vi "PID_velocity.vi"() -> ()   [LabVIEW 2014]
uses:
  <vilib>/FPGAPlugInAG/cRIO-9068/niLvFpga_Open_cRIO-9068.vi
  <vilib>/rvi/interface/common/dynamic/niFpgaDynamicAddResources.vi
  <vilib>/Utility/error.llb/Error Cluster From Error Code.vi
  <vilib>/rvi/errors/niLvFpgaAdjustHostInterfaceError.vi
  <vilib>/addons/control/pid/pid.llb/PID (DBL).vi
  <vilib>/FPGAPlugInAG/Dynamic/niLvFpga_Close_Dynamic.vi
  <vilib>/rvi/interface/nirviOpenFPGA/nirviOpenFPGA.xnode
  FPGA Bitfiles/Motortest_FPGATarget_test6auto_Jx62XASY7Q8.lvbitx
  <vilib>/rvi/interface/nirviReadWriteControl/nirviReadWriteControl.xnode
  <vilib>/rvi/interface/nirviCloseFPGA/nirviCloseFPGA.xnode
  NiFpgaLv.dll
  <vilib>/rvi/interface/Simulation/niFpgaSimulationCallBeginRW.vi
  <vilib>/addons/control/pid/NI_PID_pid.lvlib
panel:
  out "Duty Cycle":dbl[](graph)
  out "Duty Cycle":dbl(slide) scale=0.0..1.0
  out "Error":dbl(slide) scale=0.0..50.0
  out "Velocity":sgl[](graph)
  out "Duty Cycle":dbl format="%.2f"
  in  "output range":cluster{"output high":dbl, "output low":dbl}={"output high"=100.0, "output low"=-100.0} {"output low" format="%.2f"; "output high" format="%.2f"}
  in  "PID gains":T1={"proportional gain (Kc)"=0.15, "integral time (Ti, min)"=0.0002, "derivative time (Td, min)"=0.0} {"derivative time (Td, min)" format="%.4f"; "integral time (Ti, min)" format="%.4f"; "proportional gain (Kc)" format="%.4f"}
  in  "Desired Velocity":dbl=30.0 format="%.2f"
  out "Velocity [RPS]":sgl
  out "Position [Revolution]":sgl
  in  "stop":bool
  # "Error"
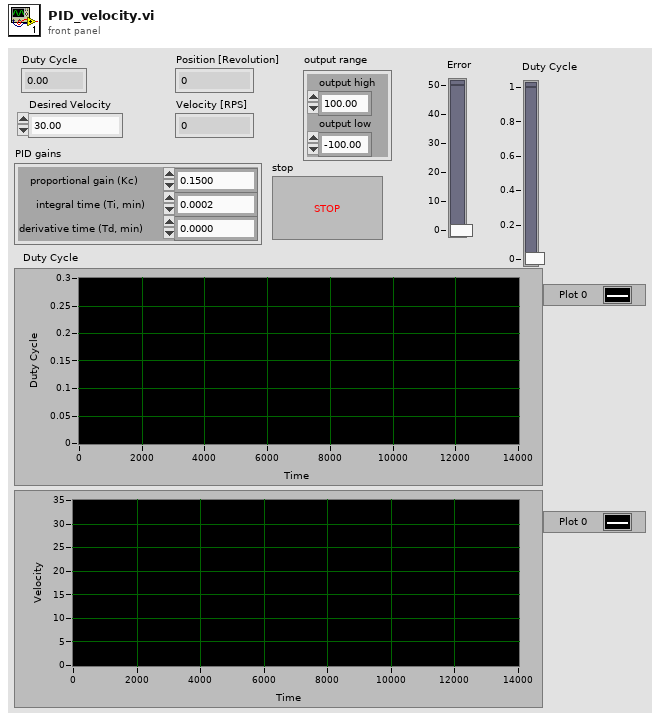
[diagram p1: front panel]
types:
  T1 = cluster{"proportional gain (Kc)":dbl, "integral time (Ti, min)":dbl, "derivative time (Td, min)":dbl}
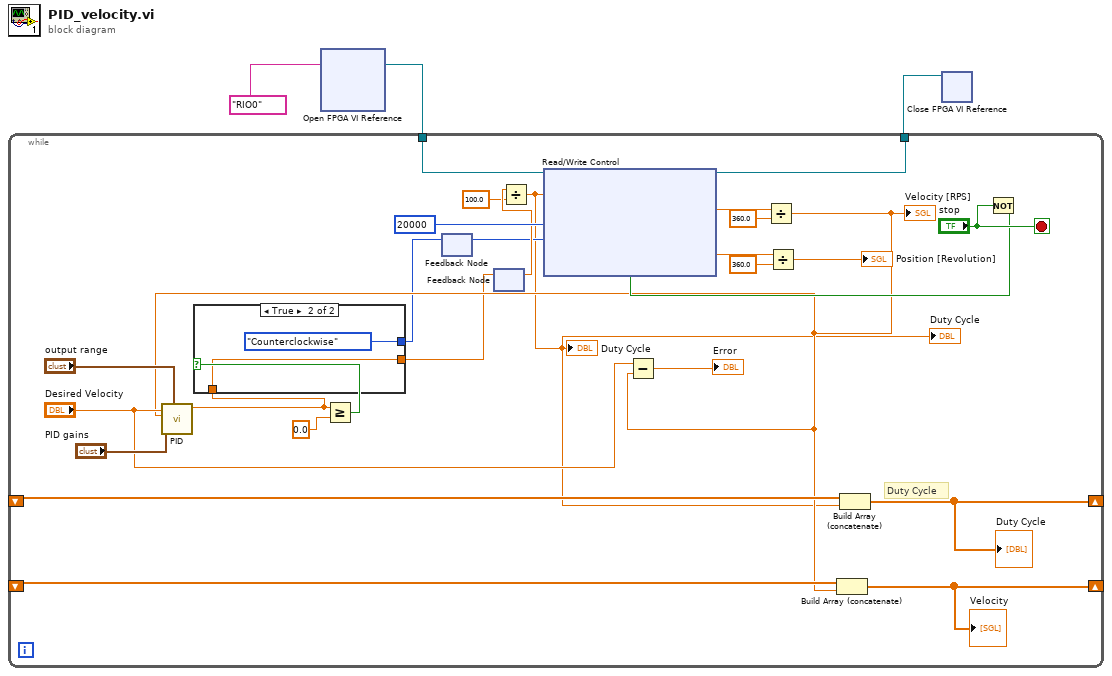
[diagram p0: block diagram]
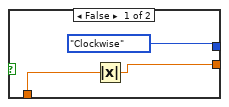
[diagram p2: hidden frame]
diagram:
  n1 = xnode "Open FPGA VI Reference"("resource name"=tag "RIO0") -> ("FPGA VI Reference Out"=w1:refnum<k20>)  [unwired: 1 in, 1 out]
  n2 = while {
    tunnel: w1 -> [w31]
    tunnel: [w30] -> w3
    shift-right: [w5] -> _
    shift-left: _ -> [w21]
    shift-right: [w6] -> _
    shift-left: _ -> [w20]
    stop <- "stop" stop-if-true
    # "Duty Cycle"
    n3 = feedback #1() -> (w8:enum8{"Clockwise", "Counterclockwise"})  [unwired: 1 in]
    n4 = feedback #2() -> (w16:dbl)  [unwired: 1 in]
    n5 = Divide(x=w16, y=100.0) -> (x/y=w4:dbl)
    "Duty Cycle" <- w4
    "Duty Cycle" <- w4
    n6 = Build Array (concatenate)(w21, w4) -> (w5:dbl[])
    "Duty Cycle" <- w5
    n7 = Not(x="stop") -> (.not. x?=w28:bool)
    n8 = xnode "Read/Write Control"("FPGA VI Reference In"=w31, "duty cycle (periods)"=w4, "Velocity Interval (uSec)"=u32 20000, "Mod1/Drive Direction"=w8, "Mod1/Motor"=w28) -> ("FPGA VI Reference Out"=w30:refnum<k20>, "Velocity (Degrees/Second)"=w18:sgl, "Position (Degrees)"=w24:sgl)  [unwired: 1 in, 1 out]
    n9 = Divide(x=w18, y=sgl 360.0) -> (x/y=w14:sgl)
    "Velocity [RPS]" <- w14
    n10 = call-poly <vilib>:"PID.vi"("output range"="output range", "PID gains"="PID gains", "process variable"=w14, "setpoint"="Desired Velocity") -> ("output"=w11:dbl)  [unwired: 6 in, 1 out]
    n11 = Greater Or Equal?(x=w11, y=0.0) -> (x >= y?=w12:bool)
    n12 = case shown="True" w12 {
      tunnel: w11 -> [w32 w36]
      tunnel: [w33 w36] -> w10
      tunnel: [enum8{"Clockwise", "Counterclockwise"}."Clockwise" ("Mod1/Drive Direction") enum8{"Clockwise", "Counterclockwise"}."Counterclockwise" ("Mod1/Drive Direction")] -> w9
      frame False {
        n13 = Absolute Value(x=w32) -> (abs(x)=w33:dbl)
      }
      frame True {
      }
    }
    n14 = feedback-in #1(w9) -> ()
    n15 = feedback-in #2(w10) -> ()
    n16 = Subtract(x="Desired Velocity", y=w14) -> (x-y=→"Error":dbl)
    n17 = Divide(x=w24, y=sgl 360.0) -> (x/y=→"Position [Revolution]":sgl)
    n18 = Build Array (concatenate)(w20, w14) -> (w6:sgl[])
    "Velocity" <- w6
  }
  n19 = xnode "Close FPGA VI Reference"("FPGA VI Reference In"=w3) -> ()  [unwired: 1 in, 1 out]
